vi "jsonClone.vi"(8 "error in (no error)":errorcluster, 10 "path":string, 11 "d in":i64) -> (0 "error out":errorcluster, 1 "clone of d":i64, 3 "d out":i64)   [LabVIEW 2016, in "JSON Document.lvclass"]
uses:
  API/JSON Document Class/JSON Document.lvclass
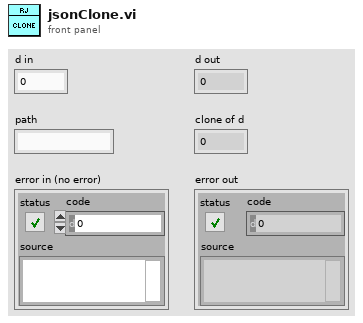
[diagram p1: front panel]
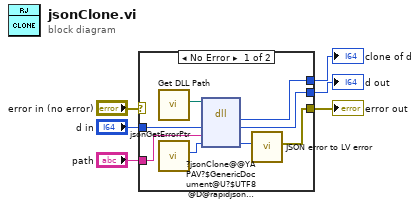
[diagram p0: block diagram]
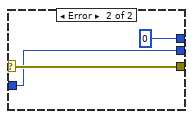
[diagram p2: hidden frame]
diagram:
  n1 = case shown="No Error" "error in (no error)" {
    selector: "error in (no error)" -> [_ w17]
    tunnel: [w11 w17] -> w6
    tunnel: "d in" -> [w10 w16]
    tunnel: [w9 w16] -> w3
    tunnel: [w8 i64 0 ("return type")] -> w2
    tunnel: "path" -> [w7 _]
    frame No Error {
      n2 = call "Get DLL Path.vi"() -> ("Path"=w14:path)  [unwired: 11 in]
      n3 = call "jsonGetErrorPtr.vi"() -> ("return type"=w13:i64)  [unwired: 10 in, 1 out]
      n4 = dll-call lib="C:/Users/tblair/Documents/Git Projects/LVrapidjson core/lvrjs/Debug/lvrjs.dll" fn="?jsonClone@@YAPAV?$GenericDocument@U?$UTF8@D@rapidjson@@V?$MemoryPoolAllocator@VCrtAllocator@rapidjson@@@2@VCrtAllocator@2@@rapidjson@@PAV12@PAD0@Z"(path in=w14, "d"=w10, "path"=w7, "jsonError"=w13) -> ("return type"=w8:i64, "d"=w9:i64, "jsonError"=w12:i64)  [unwired: 3 in, 2 out]
      n5 = call "JSON error to LV error.vi"("jsonError"=w12) -> ("error out"=w11:errorcluster)  [unwired: 10 in]
    }
    frame Error {
    }
  }
  "error out" <- w6
  "d out" <- w3
  "clone of d" <- w2
